vi "GLdrv_DATA_FORM.vi"(0 "Connection ID":T1, 5 "Format":enum16{"GBD", "CSV"}(ring), 11 "error in (no error)":errorcluster, 13 "Query(f)":bool) -> (4 "Connection ID Out":T1, 6 "Format out":enum16{"GBD", "CSV"}(ring), 15 "error out":errorcluster)   [LabVIEW 2017, in "GL860_Driver.lvlib"]
doc: "収録するデータフォーマットの設定・参照\nGBD：　バイナリ形式です。本体でのデータ再生が可能なフォーマッ\nトです。\nCSV：　テキスト形式です。主にEXCELなどで表示するためのフォー\nマットです。\n例） :DATA:FORM CSV"
uses:
  GL860_Driver.lvlib
  ConnectionID.ctl
  GLdrv_RW.ctl
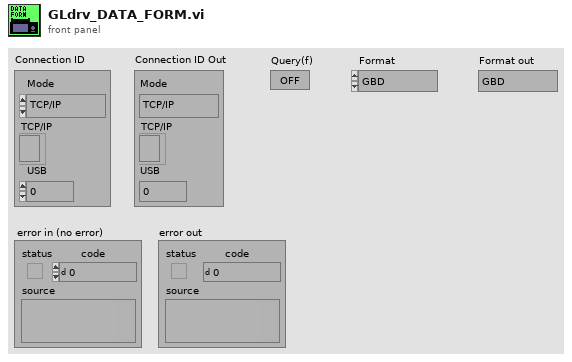
[diagram p1: front panel]
types:
  T1 = typedef "ConnectionID.ctl" = cluster{"Mode":enum16{"TCP/IP", "USB"}, "TCP/IP":refnum<k5>, "USB":i32}
  T2 = typedef "GLdrv_RW.ctl" = enum16{"Auto", "Read", "Write", "Buffer"}
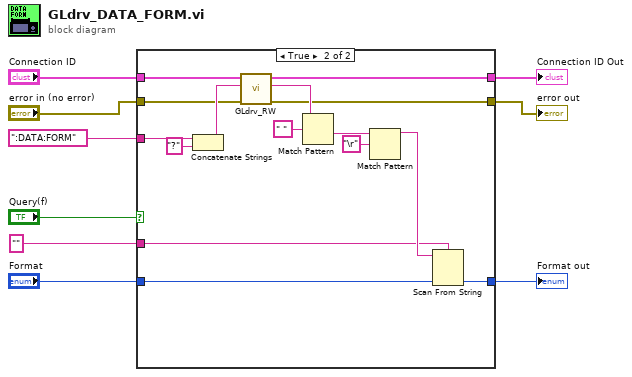
[diagram p0: block diagram]
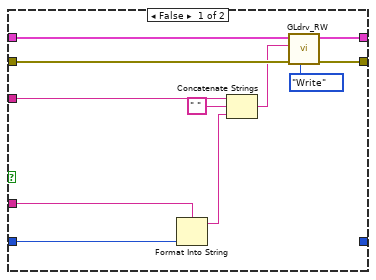
[diagram p2: hidden frame]
diagram:
  n1 = case shown="TRUE" "Query(f)" {
    tunnel: ":DATA:FORM" ("Command") -> [w20 w32]
    tunnel: [w15 w24] -> w9
    tunnel: [w17 w28] -> w8
    tunnel: "Connection ID" -> [w18 w29]
    tunnel: "error in (no error)" -> [w16 w25]
    tunnel: "Format" -> [w11 w23]
    tunnel: [_ w22] -> w1
    tunnel: "" ("Param") -> [w10 w21]
    frame False {
      n2 = Format Into String(format string=w10, w11) -> (resulting string=w12:string)  [unwired: 2 in, 1 out]
      n3 = Concatenate Strings(w20, " " ("string"), w12) -> (w14:string)
      n4 = call "GLdrv_RW.vi"("Mode(read)"=GLdrv_RW."Write", "error in (no error)"=w16, "data in"=w14, "Connection ID"=w18) -> ("error out"=w15:errorcluster, "Connection ID Out"=w17:T1)  [unwired: 3 in, 3 out]
    }
    frame True {
      n5 = Concatenate Strings(w32, "?" ("string")) -> (w27:string)
      n6 = call "GLdrv_RW.vi"("error in (no error)"=w25, "data in"=w27, "Connection ID"=w29) -> ("error out"=w24:errorcluster, "data out"=w26:string, "Connection ID Out"=w28:T1)  [unwired: 4 in, 2 out]
      n7 = Match Pattern(string=w26, regular expression=" " ("search string/char (-)")) -> (after substring=w33:string)  [unwired: 4 out]
      n8 = Match Pattern(string=w33, regular expression="\r") -> (before substring=w30:string)  [unwired: 4 out]
      n9 = Scan From String(format string=w21, input string=w30, default 1=w23) -> (output 1=w22:enum16{"GBD", "CSV"})  [unwired: 2 in, 3 out]
    }
  }
  "Connection ID Out" <- w8
  "error out" <- w9
  "Format out" <- w1
